vi "20211029_00.vi"() -> ()   [LabVIEW 2019]
panel:
  in  "Del":bool
  in  "Add":bool
  in  "Name":string
  in  "Userlist":u16(ring)
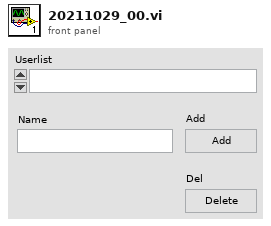
[diagram p1: front panel]
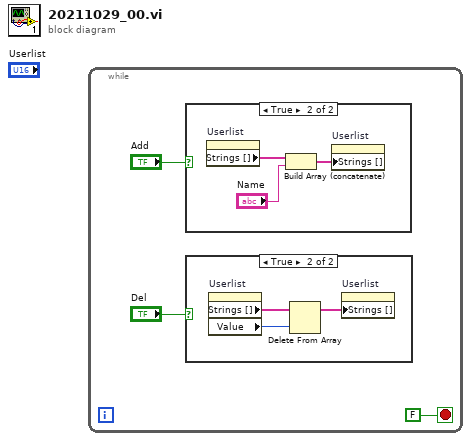
[diagram p0: block diagram]
diagram:
  n1 = while {
    stop <- FALSE stop-if-true
    n2 = case shown="True" "Add" {
      frame False {
      }
      frame True {
        n3 = property on="Userlist" class="Ring (strict)"() -> ("Strings []"=w9:string[])  [unwired: 2 in, 2 out]
        n4 = Build Array (concatenate)(w9, "Name") -> (w7:string[])
        n5 = property on="Userlist" class="Ring (strict)"("Strings []"=w7) -> ()  [unwired: 2 in, 2 out]
      }
    }
    n6 = case shown="True" "Del" {
      frame False {
      }
      frame True {
        n7 = property on="Userlist" class="Ring (strict)"() -> ("Strings []"=w6:string[], "Value"=w5:u16)  [unwired: 2 in, 2 out]
        n8 = Delete From Array(array=w6, index=w5) -> (array with subset deleted=w4:string[])  [unwired: 1 in, 1 out]
        n9 = property on="Userlist" class="Ring (strict)"("Strings []"=w4) -> ()  [unwired: 2 in, 2 out]
      }
    }
  }
